vi "AcquireWaveforms.vi"(8 "error in (no error)":errorcluster, 9 "Data Flow Maps":T11[](array[typedef]), 10 "settling time met":bool, 11 "923x Acquisition Config":T1={"Acq"=FALSE, "NumberOfModules"=0, "Dynamic FPGA VI Ref"=refnum, "KeyphasorX3"=[], "FixedSizeX32"={"EnabledChannels"=[], "Sensitivity"=[], "InputConfig"=[]}, "SamplingInfo"={"Number of Channels"=4, "Sampling Rate"=4.0, "Channels"=[], "Units"=[], "Offsets"=[]}, "Normal Mode Sample Rate"=0.0, "BlockSize (sec)"=0.0, "Samples To Read (per chan)"=0, "RunningAcquisitionLength"=0.0, "Settling Time"=0.0, "Waveform Groups"=[], "Acquisition Block Number"=0, "Device Name"="", "ValidConfig"=FALSE, "Last Dynamic Module"="", "HighPassFilterState"=[], "Low Frequency Cutoff"=[], "BurstMode"={"Acquisition Time"=0.0, "Sample Rate"=0.0}} {"HighPassFilterState"."Filter State" format="%.2f"; "HighPassFilterState"."IIR Filter Cluster"."Forward Coefficients" format="%.2f"; "HighPassFilterState"."IIR Filter Cluster"."Reverse Coefficients" format="%.2f"; "FixedSizeX32"."InputConfig" items=["AC Coupled", "DC Coupled", "IEPE AC Coupled"]}) -> (0 "error out":errorcluster, 1 "Data Flow Maps out":T11[](array[typedef]), 2 "Waveforms":waveform(sgl)[](array[waveform]), 3 "923x Acquisition Config out":T1 {"HighPassFilterState"."Filter State" format="%.2f"; "HighPassFilterState"."IIR Filter Cluster"."Forward Coefficients" format="%.2f"; "HighPassFilterState"."IIR Filter Cluster"."Reverse Coefficients" format="%.2f"; "FixedSizeX32"."InputConfig" items=["AC Coupled", "DC Coupled", "IEPE AC Coupled"]}, 4 "Pulse Positions Array":T10[](array[typedef]))   [LabVIEW 2017, in "CmsAcquisition.lvlib"]
uses:
  <vilib>/addons/InsightCM/Devices/Shared/Cms/CmsAcquisition/CmsAcquisition.lvlib
  <vilib>/addons/InsightCM/Devices/Shared/Cms/CmsAcquisition/controls/Configuration.ctl
  <vilib>/addons/InsightCM/Devices/Shared/Cms/CmsAcquisition/controls/TachometerConfig.ctl
  <vilib>/addons/InsightCM/Devices/Shared/Cms/CmsAcquisition/controls/FixedSizeArrays.ctl
  <vilib>/LabVIEW Targets/FPGA/cRIO/shared/nicrio_ModuleControls/nicrio_cRIO-9232_ConfigModeRing.ctl
  <vilib>/addons/InsightCM/Devices/Shared/Cms/cRIOWfmAcq/subVIs/RIO Wfm Cust Ctrls/rwfm_SamplingInfo.ctl
  <vilib>/addons/InsightCM/Devices/Shared/Cms/CmsAcquisition/controls/Group.ctl
  <vilib>/addons/InsightCM/Devices/Shared/Cms/CmsAcquisition/controls/Channel.ctl
  <vilib>/addons/InsightCM/Utilities/Analysis/Vibration/controls/HighPassFilterState.ctl
  <vilib>/addons/InsightCM/Devices/Shared/Cms/CmsAcquisition/controls/BurstMode.ctl
  <vilib>/addons/PointValueMap/controls/PointMap.ctl
  <vilib>/addons/InsightCM/Utilities/Analysis/Shared/controls/PulsePositions.ctl
  <vilib>/addons/PointValueMap/PointValueMap.lvlib
  <vilib>/addons/PointValueMap/subVIs/Point_Write_double.vi
  <vilib>/addons/InsightCM/Devices/Shared/Cms/cRIOWfmAcq/cRIOWfmLib.lvlib
  <vilib>/addons/InsightCM/Utilities/Analysis/Shared/AnalysisHelper.lvlib
  <vilib>/addons/InsightCM/Utilities/Analysis/Vibration/VibrationAnalysisFunctions.lvlib
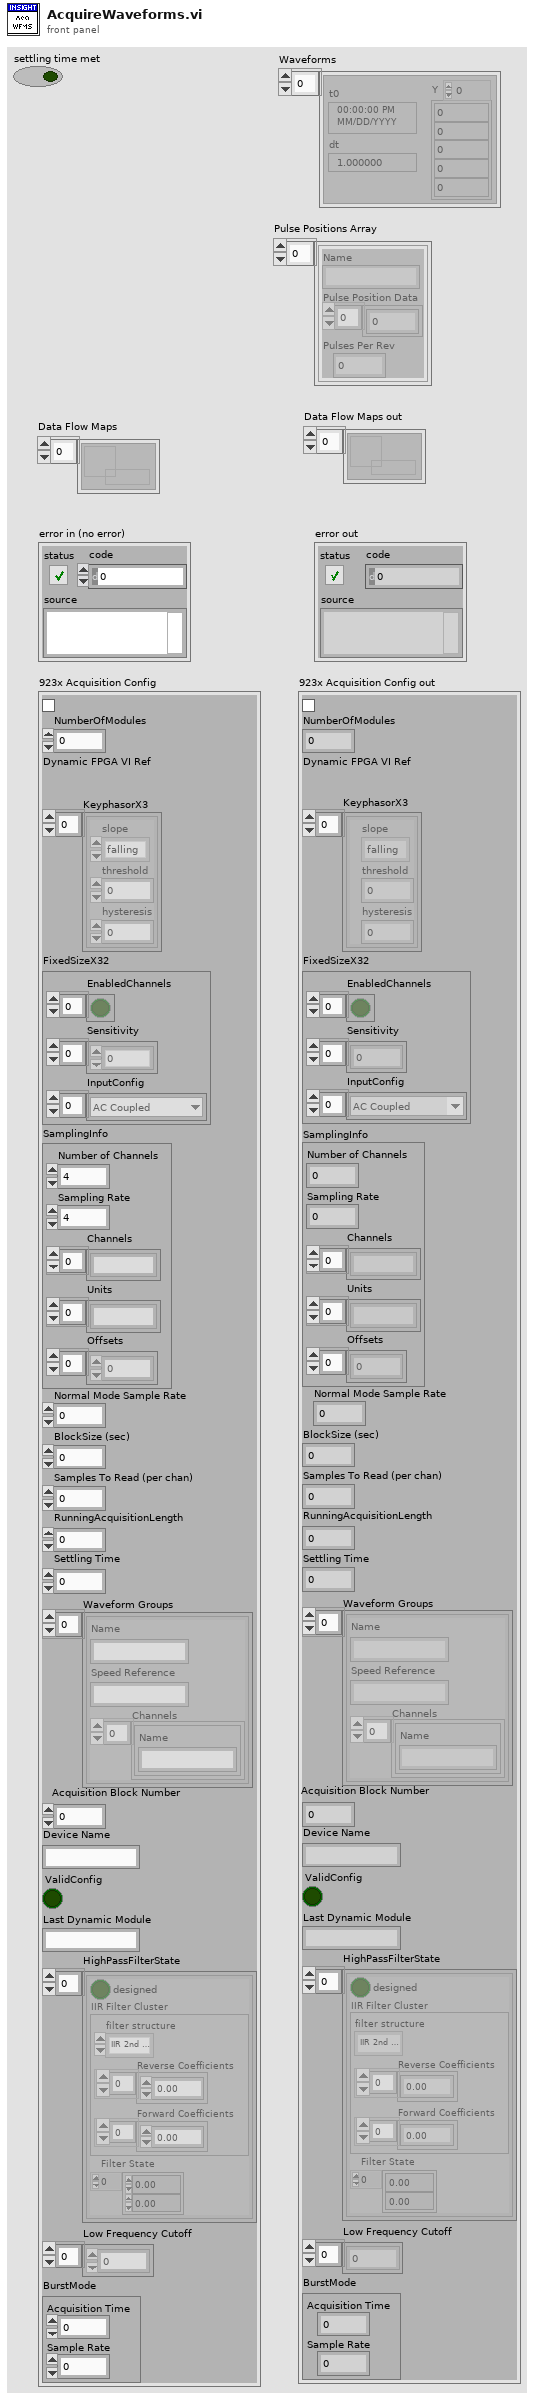
[diagram p1: front panel]
types:
  T1 = typedef "CmsAcquisition.lvlib/Configuration.ctl" = cluster{"Acq":bool, "NumberOfModules":i16, "Dynamic FPGA VI Ref":refnum<k20>, "KeyphasorX3":T2[], "FixedSizeX32":T3, "SamplingInfo":T5, "Normal Mode Sample Rate":dbl, "BlockSize (sec)":dbl, "Samples To Read (per chan)":i32, "RunningAcquisitionLength":dbl, "Settling Time":dbl, "Waveform Groups":T6[], "Acquisition Block Number":i32, "Device Name":string, "ValidConfig":bool, "Last Dynamic Module":string, "HighPassFilterState":T8[], "Low Frequency Cutoff":dbl[], "BurstMode":T9}
  T2 = typedef "CmsAcquisition.lvlib/TachometerConfig.ctl" = cluster{"slope":enum16{"falling", "rising"}, "threshold":dbl, "hysteresis":dbl}
  T3 = typedef "CmsAcquisition.lvlib/FixedSizeArrays.ctl" = cluster{"EnabledChannels":bool[], "Sensitivity":dbl[], "InputConfig":T4[]}
  T4 = typedef "nicrio_cRIO-9232_ConfigModeRing.ctl" = u8
  T5 = typedef "cRIOWfmLib.lvlib/rwfm_SamplingInfo.ctl" = cluster{"Number of Channels":i32, "Sampling Rate":dbl, "Channels":string[], "Units":string[], "Offsets":sgl[]}
  T6 = typedef "CmsAcquisition.lvlib/Group.ctl" = cluster{"Name":string, "Speed Reference":string, "Channels":T7[]}
  T7 = typedef "CmsAcquisition.lvlib/Channel.ctl" = cluster{"Name":string}
  T8 = typedef "VibrationAnalysisFunctions.lvlib/HighPassFilterState.ctl" = cluster{"designed":bool, "IIR Filter Cluster":cluster{"filter structure":enum32{"IIR 2nd Order", "IIR 4th Order"}, "Reverse Coefficients":dbl[], "Forward Coefficients":dbl[]}, "Filter State":dbl[]}
  T9 = typedef "CmsAcquisition.lvlib/BurstMode.ctl" = cluster{"Acquisition Time":dbl, "Sample Rate":dbl}
  T10 = typedef "AnalysisHelper.lvlib/PulsePositions.ctl" = cluster{"Name":string, "Pulse Position Data":dbl[], "Pulses Per Rev":i32}
  T11 = typedef "PointValueMap.lvlib/PointMap.ctl" = refnum<data-value>
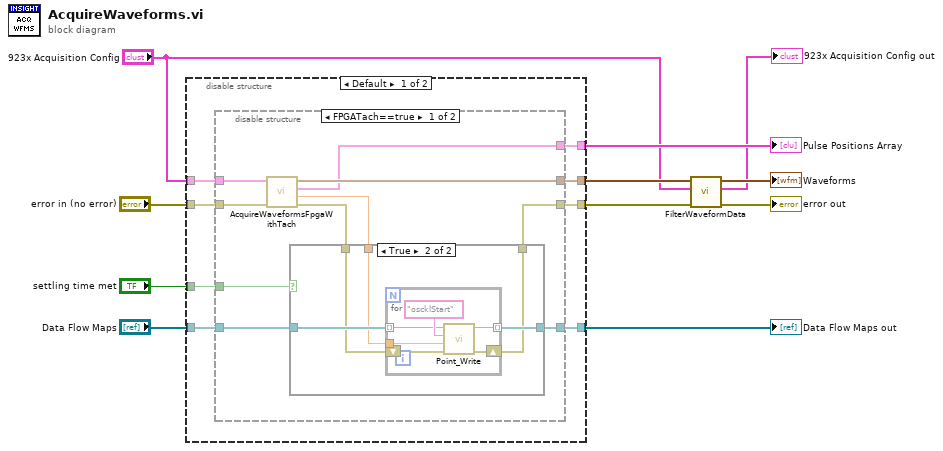
[diagram p0: block diagram]
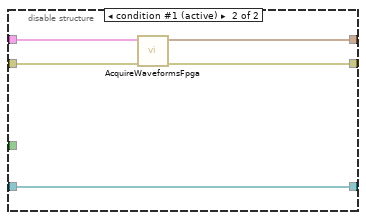
[diagram p3: hidden frame]
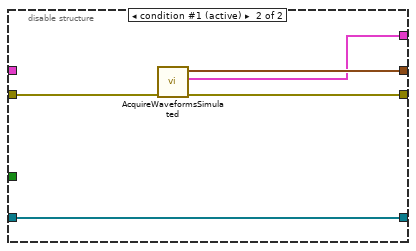
[diagram p4: hidden frame]
diagram:
  n1 = disable-structure shown="Default" {
    disable-tunnel: "error in (no error)" -> [w19 w52]
    disable-tunnel: [w18 w51] -> w4
    disable-tunnel: [w17 w50] -> w5
    disable-tunnel: [w16 w49] -> w10
    disable-tunnel: "Data Flow Maps" -> [w15 w48]
    disable-tunnel: [w14 w48] -> w11
    disable-tunnel: "923x Acquisition Config" -> [w13 _]
    disable-tunnel: "settling time met" -> [w12 _]
    frame condition #0 {
      n2 = disable-structure shown="FPGATach==true" {
        disable-tunnel: w19 -> [w28 w47]
        disable-tunnel: [w21 w46] -> w17
        disable-tunnel: [w29 w45] -> w18
        disable-tunnel: [w27 _] -> w16
        disable-tunnel: w15 -> [w26 w44]
        disable-tunnel: [w24 w44] -> w14
        disable-tunnel: w13 -> [w23 w43]
        disable-tunnel: w12 -> [w20 _]
        frame condition #0 {
          n3 = call <vilib>:"AcquireWaveformsFpgaWithTach.vi"("error in (no error)"=w28, "923x Acquisition Config"=w23) -> ("error out"=w22:errorcluster, "OSClkStart"=w25:dbl, "Pulse Positions Array"=w27:T10[], "Waveforms"=w29:waveform(sgl)[])  [unwired: 6 in]
          n4 = case shown="True" w20 {
            tunnel: w26 -> [w30 w36]
            tunnel: w25 -> [_ w35]
            tunnel: [w30 w34] -> w24
            tunnel: w22 -> [w31 w33]
            tunnel: [w31 w32] -> w21
            frame False {
            }
            frame True {
              n5 = for {
                tunnel: w36 -> [w41] mode=indexing
                tunnel: w35 -> [w40]
                tunnel: [w38] -> w34 mode=indexing
                shift-right: [w37] -> w32
                shift-left: w33 -> [w39]
                n6 = call-poly <vilib>:"Point_Write.vi"("Error In"=w39, "Value"=w40, "Tag"="oscklStart", "Map"=w41) -> ("Error Out"=w37:errorcluster, "Map Out"=w38:T11)  [unwired: 6 in]
              }
            }
          }
        }
        frame condition #1 (active) {
          n7 = call <vilib>:"AcquireWaveformsFpga.vi"("error in (no error)"=w47, "923x Acquisition Config"=w43) -> ("error out"=w46:errorcluster, "Waveforms"=w45:waveform(sgl)[])  [unwired: 8 in]
        }
      }
    }
    frame condition #1 (active) {
      n8 = call <vilib>:"AcquireWaveformsSimulated.vi"("error in (no error)"=w52) -> ("error out"=w50:errorcluster, "simulated pulse position array"=w49:T10[], "simulated waveforms"=w51:waveform(sgl)[])  [unwired: 8 in]
    }
  }
  "Data Flow Maps out" <- w11
  "Pulse Positions Array" <- w10
  n9 = call <vilib>:"FilterWaveformData.vi"("error in (no error)"=w5, "923x Acquisition Config"="923x Acquisition Config", "waveforms in"=w4) -> ("error out"=→"error out":errorcluster, "923x Acquisition Config out"=→"923x Acquisition Config out":T1, "waveforms out"=→"Waveforms":waveform(sgl)[])  [unwired: 6 in]
